vi "Fast_slow loop.vi"() -> ()   [LabVIEW 2020]
panel:
  in  "Stop Loop 2":bool
  out "Loop 2 Iteration Rate (Hz)":dbl
  out "Loop 1 Iteration Rate (Hz)":dbl
  in  "Stop Loop 1":bool
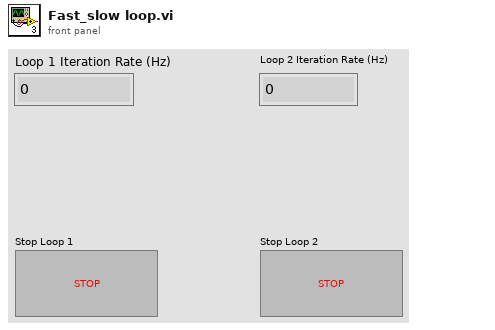
[diagram p1: front panel]
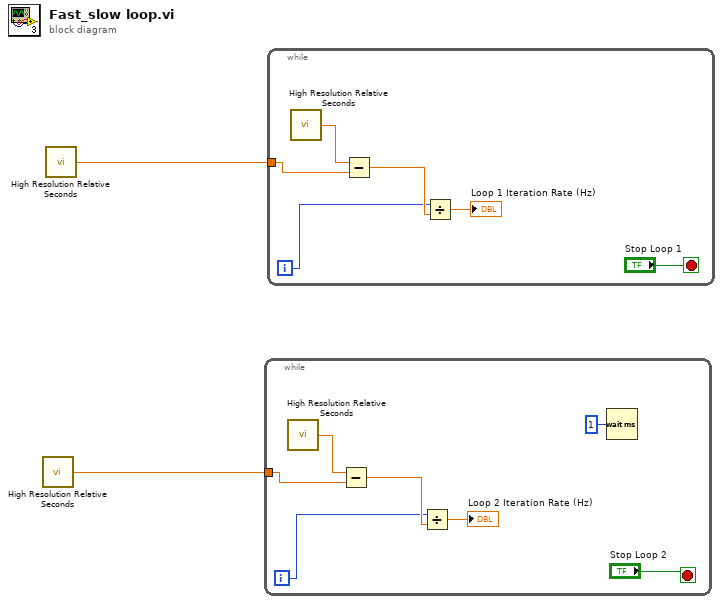
[diagram p0: block diagram]
diagram:
  n1 = call <vilib>:"High Resolution Relative Seconds.vi"() -> ("relative seconds"=w2:dbl)
  n2 = call <vilib>:"High Resolution Relative Seconds.vi"() -> ("relative seconds"=w1:dbl)
  n3 = while {
    tunnel: w2 -> [w7]
    i -> [w6]
    stop <- "Stop Loop 2" stop-if-true
    n4 = call <vilib>:"High Resolution Relative Seconds.vi"() -> ("relative seconds"=w8:dbl)
    n5 = Subtract(x=w8, y=w7) -> (x-y=w9:dbl)
    n6 = Divide(x=w6, y=w9) -> (x/y=→"Loop 2 Iteration Rate (Hz)":dbl)
    n7 = Wait (ms)(milliseconds to wait=u32 1) -> ()  [unwired: 1 out]
  }
  n8 = while {
    tunnel: w1 -> [w12]
    i -> [w11]
    stop <- "Stop Loop 1" stop-if-true
    n9 = call <vilib>:"High Resolution Relative Seconds.vi"() -> ("relative seconds"=w13:dbl)
    n10 = Subtract(x=w13, y=w12) -> (x-y=w14:dbl)
    n11 = Divide(x=w11, y=w14) -> (x/y=→"Loop 1 Iteration Rate (Hz)":dbl)
  }
